vi "Data.Evaluate Status Comparing Limit of Result Numeric.vi"(9 "Limit Def":T2, 10 "Value":dbl) -> (1 "Desc":string, 2 "Status":T1 items=["LOG", "PASS", "FAIL", "ERROR"])   [LabVIEW 2024, in "EQMF.lvlib" / "Data.lvlib"]
uses:
  Data.lvlib
  TypeDefs/Data.Result Numeric Limit Type with Limits.ctl
  TypeDefs/Data.Result Numeric Limit Type.ctl
  TypeDefs/Data.Result Item Status.ctl
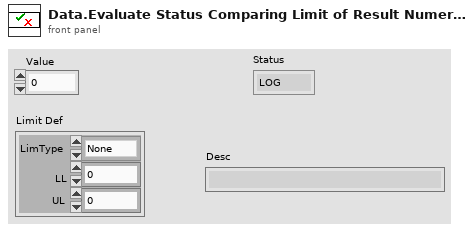
[diagram p1: front panel]
types:
  T1 = typedef "EQMF.lvlib/Data.lvlib/Data.Result Item Status.ctl" = i32
  T2 = typedef "EQMF.lvlib/Data.lvlib/Data.Result Numeric Limit Type with Limits.ctl" = cluster{"LimType":T3, "LL":dbl, "UL":dbl}
  T3 = typedef "EQMF.lvlib/Data.lvlib/Data.Result Numeric Limit Type.ctl" = enum16{"None", "EQ", "NE", "GT", "LT", "GE", "LE", "GTLT", "GELE", "GELT", "GTLE", "LTGT", "LEGE", "LEGT", "LTGE"}
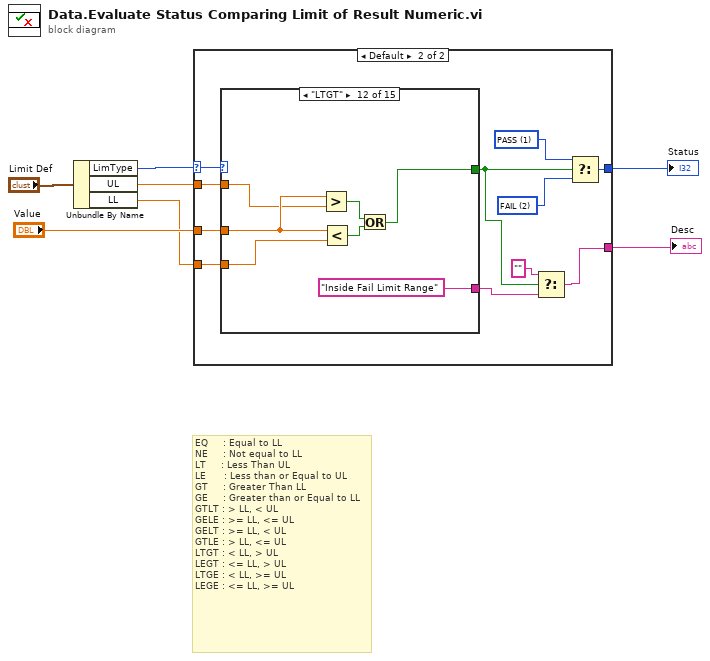
[diagram p0: block diagram]
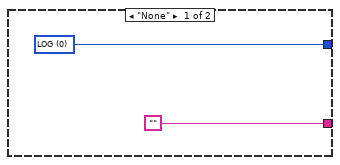
[diagram p2: hidden frame]
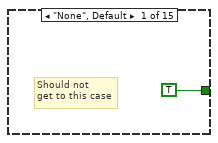
[diagram p3: hidden frame]
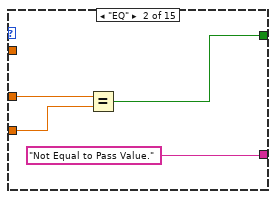
[diagram p4: hidden frame]
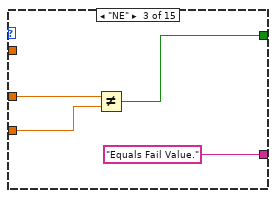
[diagram p5: hidden frame]
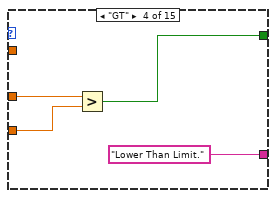
[diagram p6: hidden frame]
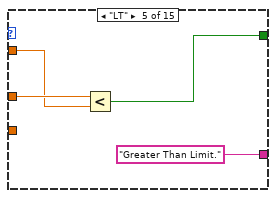
[diagram p7: hidden frame]
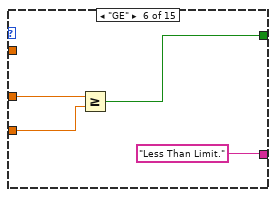
[diagram p8: hidden frame]
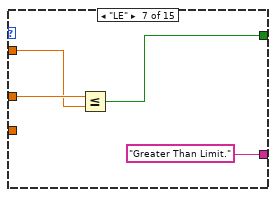
[diagram p9: hidden frame]
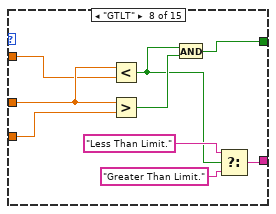
[diagram p10: hidden frame]
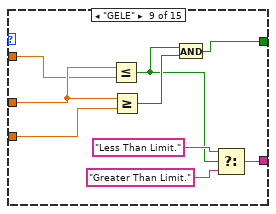
[diagram p11: hidden frame]
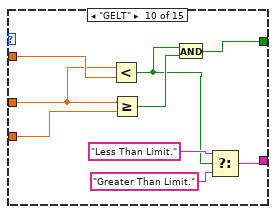
[diagram p12: hidden frame]
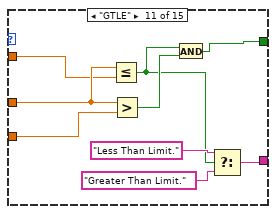
[diagram p13: hidden frame]
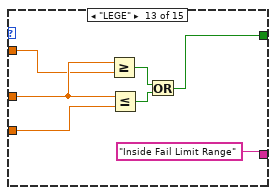
[diagram p14: hidden frame]
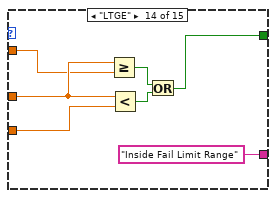
[diagram p15: hidden frame]
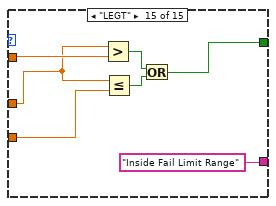
[diagram p16: hidden frame]
diagram:
  # "EQ     : Equal to LL\nNE     : Not equal to LL\nLT     : Less Than UL\nLE      : Less than or Equal to UL\nGT     : Greater Than LL\nGE     : Greater than or Equal to LL\nGTLT : > LL, < UL\nGELE : >= LL, <= UL\nGELT : >= LL, < UL\nGTLE : > LL, <= UL\nLTGT : < LL, > UL\nLEGT : <= LL, > UL\nLTGE : < LL, >= UL\nLEGE : <= LL, >= UL"
  n1 = Unbundle By Name("Limit Def") -> ("LimType"=w3:T3, "UL"=w5:dbl, "LL"=w4:dbl)
  n2 = case shown="Default" w3 {
    selector: w3 -> [_ w17]
    tunnel: "Value" -> [_ w20]
    tunnel: w5 -> [_ w19]
    tunnel: w4 -> [_ w18]
    tunnel: [w9 w14] -> w2
    tunnel: ["" w13] -> w1
    frame "None" {
      w9 = T1 0 items=["LOG", "PASS", "FAIL", "ERROR"] ("Status")
    }
    frame Default {
      w16 = T1 2 items=["LOG", "PASS", "FAIL", "ERROR"] ("Status")
      w15 = T1 1 items=["LOG", "PASS", "FAIL", "ERROR"] ("Status")
      n3 = case shown="\"LTGT\"" w17 {
        tunnel: w19 -> [_ _ _ _ w35 _ w44 w51 w62 w72 w80 w87 w94 w101 w107]
        tunnel: w20 -> [_ w25 w29 w33 w37 w41 w45 w54 w63 w70 w81 w88 w95 w102 w106]
        tunnel: w18 -> [_ w24 w28 w32 _ w40 _ w53 w61 w71 w79 w86 w93 w100 w105]
        tunnel: [TRUE w23 w27 w31 w36 w39 w43 w50 w59 w68 w77 w83 w90 w97 w104] -> w11
        tunnel: [_ "Not Equal to Pass Value." "Equals Fail Value." "Lower Than Limit." "Greater Than Limit." "Less Than Limit." "Greater Than Limit." w47 w56 w65 w74 "Inside Fail Limit Range" "Inside Fail Limit Range" "Inside Fail Limit Range" "Inside Fail Limit Range"] -> w12
        frame "None", Default {
          # "Should not\nget to this case"
        }
        frame "EQ" {
          n4 = Equal?(x=w25, y=w24) -> (x = y?=w23:bool)
        }
        frame "NE" {
          n5 = Not Equal?(x=w29, y=w28) -> (x != y?=w27:bool)
        }
        frame "GT" {
          n6 = Greater?(x=w33, y=w32) -> (0:w31:bool)
        }
        frame "LT" {
          n7 = Less?(x=w37, y=w35) -> (x < y?=w36:bool)
        }
        frame "GE" {
          n8 = Greater Or Equal?(x=w41, y=w40) -> (x >= y?=w39:bool)
        }
        frame "LE" {
          n9 = Less Or Equal?(x=w45, y=w44) -> (x <= y?=w43:bool)
        }
        frame "GTLT" {
          n10 = Less?(x=w54, y=w51) -> (x < y?=w46:bool)
          n11 = Greater?(x=w54, y=w53) -> (0:w52:bool)
          n12 = And(x=w46, y=w52) -> (x .and. y?=w50:bool)
          n13 = Select(t="Less Than Limit.", s=w46, f="Greater Than Limit.") -> (s? t:f=w47:string)
        }
        frame "GELE" {
          n14 = Less Or Equal?(x=w63, y=w62) -> (x <= y?=w55:bool)
          n15 = Greater Or Equal?(x=w63, y=w61) -> (x >= y?=w60:bool)
          n16 = And(x=w55, y=w60) -> (x .and. y?=w59:bool)
          n17 = Select(t="Less Than Limit.", s=w55, f="Greater Than Limit.") -> (s? t:f=w56:string)
        }
        frame "GELT" {
          n18 = Less?(x=w70, y=w72) -> (x < y?=w64:bool)
          n19 = Greater Or Equal?(x=w70, y=w71) -> (x >= y?=w69:bool)
          n20 = And(x=w64, y=w69) -> (x .and. y?=w68:bool)
          n21 = Select(t="Less Than Limit.", s=w64, f="Greater Than Limit.") -> (s? t:f=w65:string)
        }
        frame "GTLE" {
          n22 = Less Or Equal?(x=w81, y=w80) -> (x <= y?=w73:bool)
          n23 = Greater?(x=w81, y=w79) -> (0:w78:bool)
          n24 = And(x=w73, y=w78) -> (x .and. y?=w77:bool)
          n25 = Select(t="Less Than Limit.", s=w73, f="Greater Than Limit.") -> (s? t:f=w74:string)
        }
        frame "LTGT" {
          n26 = Greater?(x=w88, y=w87) -> (0:w85:bool)
          n27 = Less?(x=w88, y=w86) -> (x < y?=w84:bool)
          n28 = Or(x=w85, y=w84) -> (x .or. y?=w83:bool)
        }
        frame "LEGE" {
          n29 = Greater Or Equal?(x=w95, y=w94) -> (x >= y?=w92:bool)
          n30 = Less Or Equal?(x=w95, y=w93) -> (x <= y?=w91:bool)
          n31 = Or(x=w92, y=w91) -> (x .or. y?=w90:bool)
        }
        frame "LTGE" {
          n32 = Greater Or Equal?(x=w102, y=w101) -> (x >= y?=w99:bool)
          n33 = Less?(x=w102, y=w100) -> (x < y?=w98:bool)
          n34 = Or(x=w99, y=w98) -> (x .or. y?=w97:bool)
        }
        frame "LEGT" {
          n35 = Greater?(x=w106, y=w107) -> (0:w109:bool)
          n36 = Less Or Equal?(x=w106, y=w105) -> (x <= y?=w108:bool)
          n37 = Or(x=w109, y=w108) -> (x .or. y?=w104:bool)
        }
      }
      n38 = Select(t="", s=w11, f=w12) -> (s? t:f=w13:string)
      n39 = Select(t=w15, s=w11, f=w16) -> (s? t:f=w14:T1)
    }
  }
  "Status" <- w2
  "Desc" <- w1
